vi "Create emibin top Header.vi"(5 "File type Std(0)":u8 format="%.0x", 7 "File type ID":u16=1 format="%.0x", 9 "File type Version":u8 format="%.0x", 11 "error in (no error)":errorcluster) -> (8 "bin ID header":T1={"Fixed code"=255158202, "File type Std"=0, "File type ID"=1, "File type Version"=0} {"File type Std" format="%.0x"; "Fixed code" format="%.0x"; "File type ID" format="%.0x"; "File type Version" format="%.0x"}, 15 "error out":errorcluster)   [LabVIEW 2011]
uses:
  Header.ctl
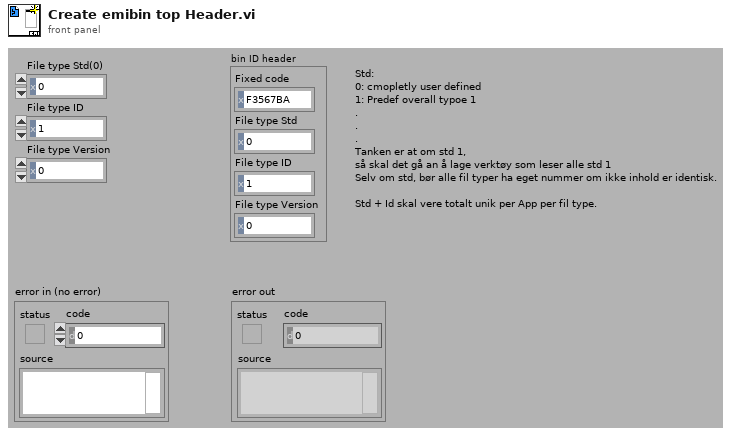
[diagram p1: front panel]
types:
  T1 = typedef "Header.ctl" = cluster{"Fixed code":u32, "File type Std":u8, "File type ID":u16, "File type Version":u8}
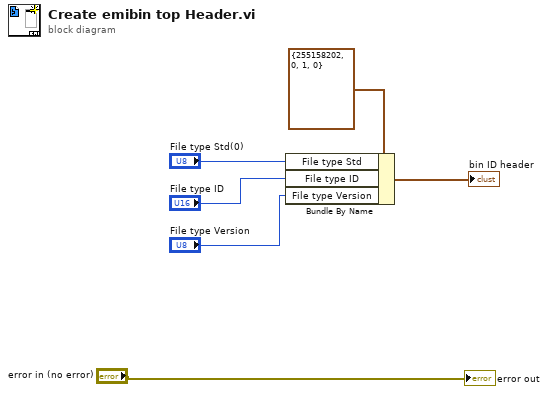
[diagram p0: block diagram]
diagram:
  n1 = Bundle By Name(cluster=T1 {"Fixed code"=255158202, "File type Std"=0, "File type ID"=1, "File type Version"=0} ("bin ID header"), "File type Std"="File type Std(0)", "File type ID"="File type ID", "File type Version"="File type Version") -> (→"bin ID header":T1)
  "error out" <- "error in (no error)"
